vi "Acquire_Hardware.vi"(8 "error in (no error)":errorcluster, 11 "FROG in":refnum<class "FROG.lvclass">) -> (0 "error out":errorcluster, 2 "new command":string, 3 "FROG out":refnum<class "FROG.lvclass">)   [LabVIEW 2020, in "FROG.lvclass"]
uses:
  FROG.lvclass
  FROG.lvclass/FROG.ctl
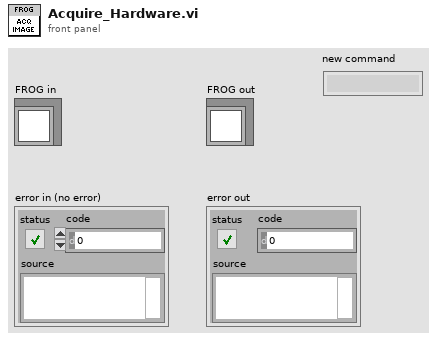
[diagram p1: front panel]
types:
  T1 = typedef "IMAQ Image.ctl" = refnum<image>
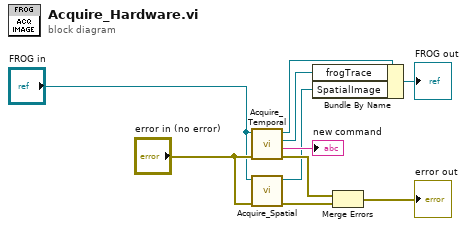
[diagram p0: block diagram]
diagram:
  n1 = call "Acquire_Temporal.vi"("error in (no error)"="error in (no error)", "FROG in"="FROG in") -> ("error out"=w8:errorcluster, "String"=→"new command":string, "frogTrace"=w5:T1, "FROG out"=w3:refnum<class "FROG.lvclass">)  [unwired: 6 in]
  n2 = call "Acquire_Spatial.vi"("error in (no error)"="error in (no error)", "FROG in"="FROG in") -> ("error out"=w9:errorcluster, "frogTrace"=w4:T1)  [unwired: 8 in]
  n3 = Bundle By Name(cluster=w3, "frogTrace"=w5, "SpatialImage"=w4) -> (→"FROG out":refnum<class "FROG.lvclass">)
  n4 = Merge Errors(w8, w9) -> (→"error out":errorcluster)
